vi "publisher tests Writer 2.vi"() -> ()   [LabVIEW 2018]
uses:
  publisher action.ctl
panel:
  out "number":dbl
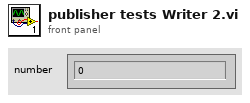
[diagram p1: front panel]
types:
  T1 = typedef "publisher action.ctl" = enum16{"set", "get", "init", "check"}
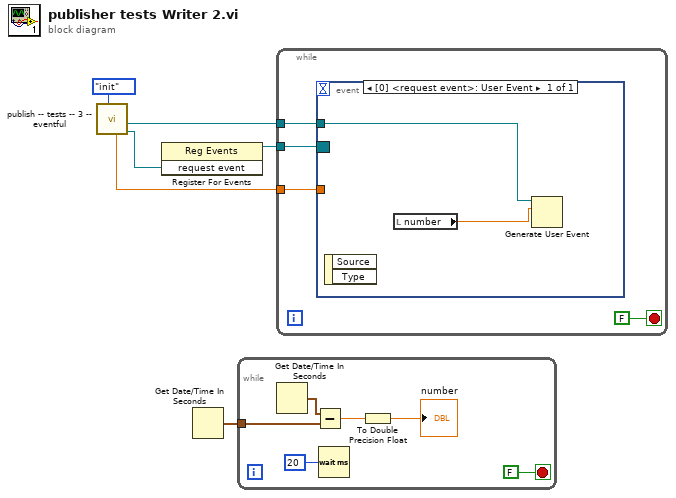
[diagram p0: block diagram]
diagram:
  n1 = call "publish -- tests -- 3 -- eventful.vi"("publisher action"=publisher_action."init") -> ("request event"=w5:refnum<user-event>, "response event"=w4:refnum<user-event>, "response type"=w1:dbl)  [unwired: 7 in, 1 out]
  n2 = register-events(w5) -> (reference out=w6:refnum<event-registration>)  [unwired: 2 in, 1 out]
  n3 = Get Date/Time In Seconds() -> (seconds since 1Jan1904=w2:timestamp)
  n4 = while {
    tunnel: w2 -> [w9]
    stop <- FALSE stop-if-true
    n5 = Get Date/Time In Seconds() -> (seconds since 1Jan1904=w11:timestamp)
    n6 = Subtract(x=w11, y=w9) -> (x-y=w12:dbl)
    n7 = Wait (ms)(milliseconds to wait=u32 20) -> ()  [unwired: 1 out]
    n8 = To Double Precision Float(number=w12) -> (double precision float=→"number":dbl)
  }
  n9 = while {
    tunnel: w6 -> [w15]
    tunnel: w4 -> [w14]
    tunnel: w1 -> [w13]
    stop <- FALSE stop-if-true
    n10 = event shown="[0] <request event>: User Event" {
      selector: w15 -> [_]
      dyn-events: _ -> [_]
      timeout: _ -> [_]
      tunnel: w14 -> [w18]
      tunnel: w13 -> [_]
      event User Event {
        n11 = event-data() -> ()  [unwired: 1 in, 2 out]
        n12 = local read "number"() -> (w17:dbl)
        n13 = Generate User Event(user event=w18, event data cluster=w17) -> ()  [unwired: 2 in, 2 out]
      }
    }
  }
